vi "plate tap.vi"() -> ()   [LabVIEW 2014]
panel:
  in  "Hold Time (frames)":i32
  in  "ISI  (frames)":i32
  in  "Trials Per Voltage":i32
  in  "Array":dbl[](array[numeric])
  in  "Min Voltage":dbl
  out "Frames":i32
  in  "Transfer and Run Date Folder After Experiment":bool
  in  "SSH user name":string
  in  "SSH password":string
  in  "Wait before recording (s)":dbl
  in  "Tags":string
  in  "Start Recording":bool
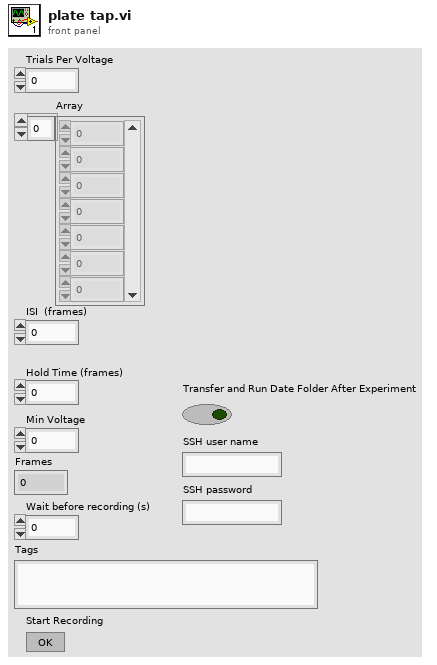
[diagram p1: front panel]
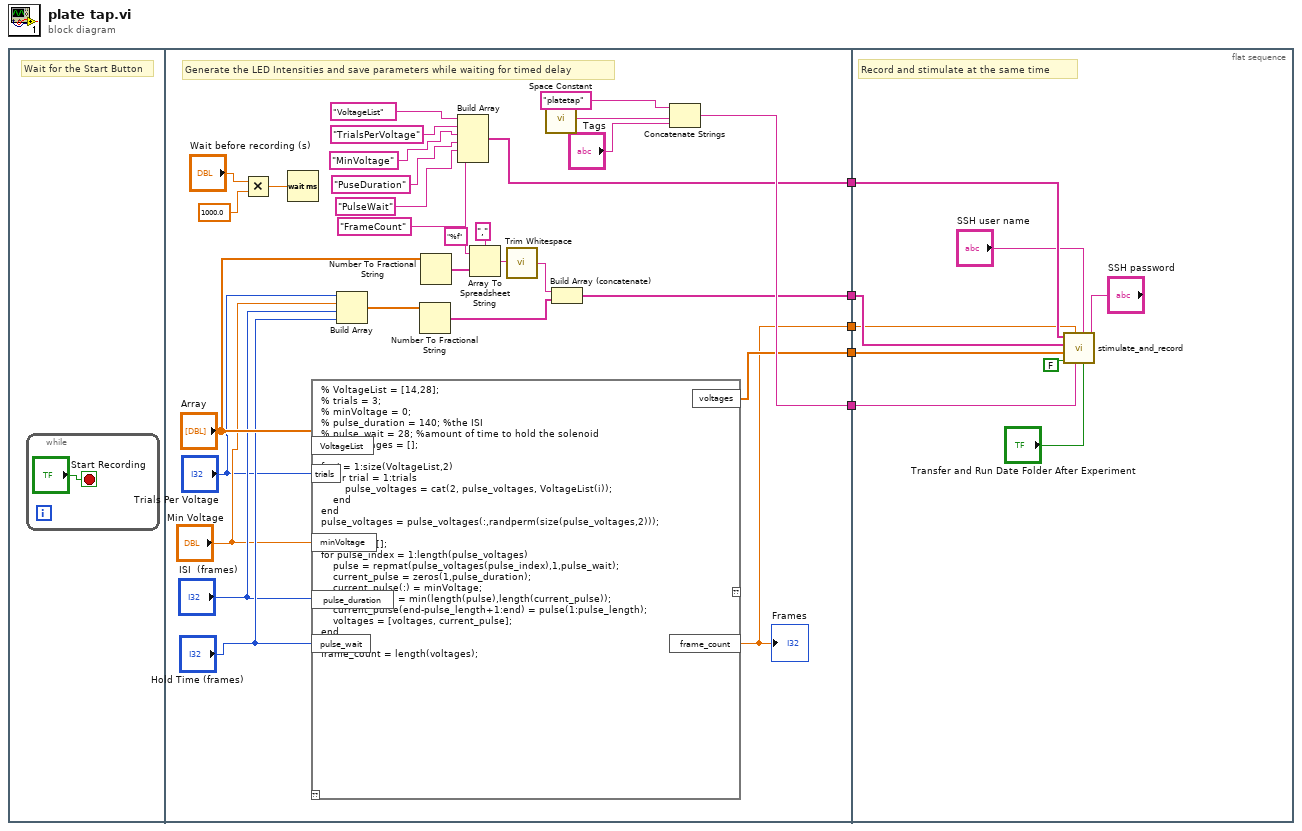
[diagram p0: block diagram]
diagram:
  n1 = flat-sequence {
    tunnel: [w32] -> w5
    tunnel: [w16] -> w4
    tunnel: [w26] -> w3
    tunnel: [w8] -> w2
    tunnel: [w7] -> w1
    tunnel: w5 -> [w44]
    tunnel: w4 -> [w42]
    tunnel: w3 -> [w38]
    tunnel: w2 -> [w37]
    tunnel: w1 -> [w36]
    frame #0 {
      # "Wait for the Start Button"
      n2 = while {
        stop <- "Start Recording" stop-if-true
      }
    }
    frame #1 {
      # "Generate the LED Intensities and save parameters while waiting for timed delay"
      n3 = Multiply(x="Wait before recording (s)", y=1000.0) -> (x*y=w30:dbl)
      n4 = Wait (ms)(milliseconds to wait=w30) -> ()  [unwired: 1 out]
      n5 = script code="% VoltageList = [14,28];\n% trials = 3;\n% minVoltage = 0;\n% pulse_duration = 140; %the ISI\n% pulse_wait = 28; %amount of time to hold the solenoid\npulse_voltages = [];\n\nfor i = 1:size(VoltageList,2)\n    for trial = 1:trials\n        pulse_voltages = cat(2, pulse_voltages, VoltageList(i));\n    end\nend\npulse_voltages = pulse_voltages(:,randperm(size(pulse_voltages,2)));\n\nvoltages = [];\nfor pulse_index = 1:length(pulse_voltages)\n    pulse = repmat(pulse_voltages(pulse_index),1,pulse_wait);\n    current_pulse = zeros(1,pulse_duration);\n    current_pulse(:) = minVoltage;\n    pulse_length = min(length(pulse),length(current_pulse));\n    current_pulse(end-pulse_length+1:end) = pulse(1:pulse_length);\n    voltages = [voltages, current_pulse];\nend\n\nframe_count = length(voltages);"("pulse_duration"="ISI  (frames)", "trials"="Trials Per Voltage", "minVoltage"="Min Voltage", "VoltageList"="Array", "pulse_wait"="Hold Time (frames)") -> ("voltages"=w8:dbl[], "frame_count"=w7:dbl)  [unwired: 1 in, 1 out]
      "Frames" <- w7
      n6 = Build Array("Trials Per Voltage", "Min Voltage", "ISI  (frames)", "Hold Time (frames)") -> (w15:dbl[])
      n7 = Number To Fractional String(number=w15) -> (F-format string=w27:string[])  [unwired: 3 in]
      n8 = Number To Fractional String(number="Array") -> (F-format string=w14:string[])  [unwired: 3 in]
      n9 = Build Array("VoltageList", "TrialsPerVoltage", "MinVoltage", "PuseDuration", "PulseWait", "FrameCount") -> (w16:string[])
      n10 = Array To Spreadsheet String(delimiter (Tab)=",", array=w14, 3:"%f") -> (spreadsheet string=w24:string)
      n11 = call <vilib>:"Trim Whitespace.vi"("string"=w24) -> ("trimmed string"=w23:string)  [unwired: 1 in]
      n12 = call <vilib>:"Space Constant.vi"() -> ("String"=w34:string)
      n13 = Build Array (concatenate)(w23, w27) -> (w26:string[])
      n14 = Concatenate Strings("platetap", w34, "Tags") -> (w32:string)
    }
    frame #2 {
      # "Record and stimulate at the same time"
      n15 = call "stimulate_and_record.vi"("SSH password"="SSH password", "Transfer and Run Date Folder After Experiment"="Transfer and Run Date Folder After Experiment", "SSH user name"="SSH user name", "Tags"=w44, "Frames"=w36, "Convert Power to Voltage"=FALSE, "voltages/power"=w37, "parameters"=w38, "parameters headers"=w42) -> ()  [unwired: 3 in]
    }
  }
